vi "total.vi"() -> ()   [LabVIEW 2018]
panel:
  out "解码":i8[](array[numeric])
  in  "n":dbl=3.0
  out "编码":i8[](array[numeric])
  in  "输入":i8[](array[numeric])
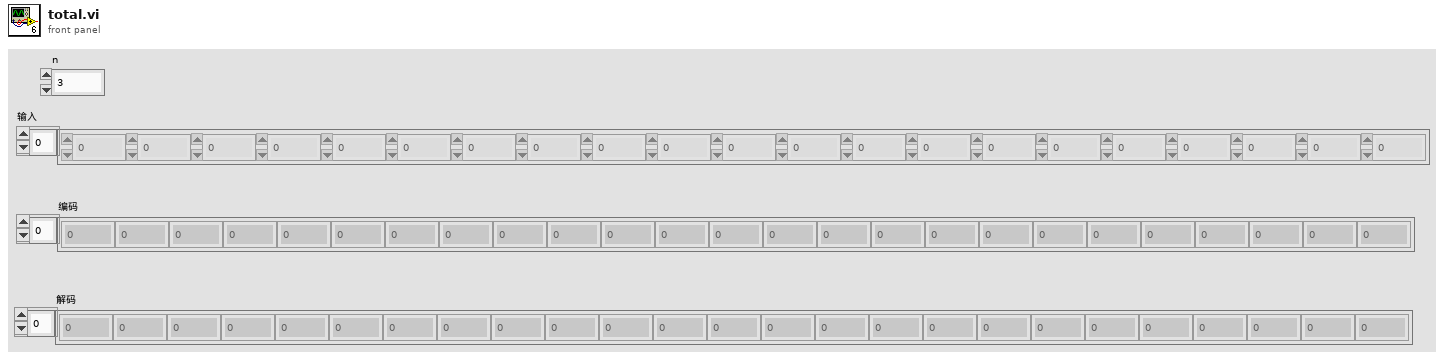
[diagram p1: front panel]
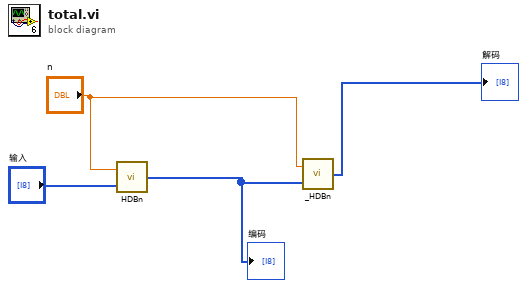
[diagram p0: block diagram]
diagram:
  n1 = call "HDBn.vi"("输入"="输入", "n"="n") -> ("输出"=w3:i8[])
  "编码" <- w3
  n2 = call "_HDBn.vi"("输入"=w3, "n"="n") -> ("输出"=→"解码":i8[])
